vi "Extract_Hex_From_String_Delimited_With_Bytes_LV2015.vi"(8 "error in (no error)":errorcluster, 11 "String":string="1234 56 7 8 9A BC DEF1\nabcdefghijklmnopqrstuvwxyz1234567890\n\nasdfjlkasjdf;lk ajsdovj 239845uj sdklfhjg98bn248vg 9mufy gfalkjdfn" caption="HexString with or without delimitation") -> (0 "error out":errorcluster, 3 "Extracted Hex with delimitation at every byte":string="12 34 56 78 9A BC DE F1 AB CD EF 12 34 56 78 90 AD FA DF AD 23 98 45 DF 98 B2 48 9F FA DF" caption="HexByte delimited string")   [LabVIEW 2015]
panel:
  # "Connector Pane"
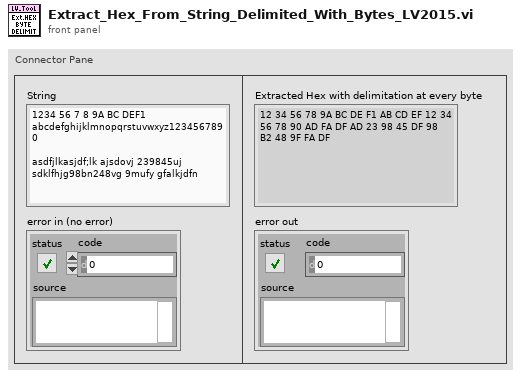
[diagram p1: front panel]
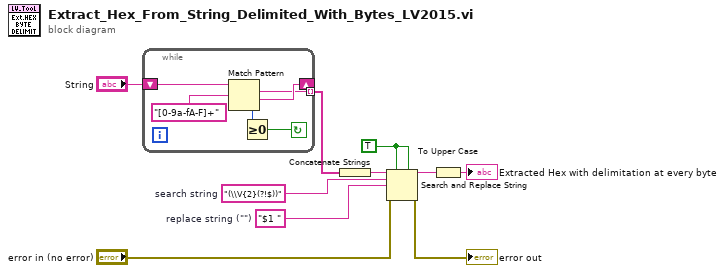
[diagram p0: block diagram]
diagram:
  w7 = TRUE ("replace all? (F)")
  w9 = "$1 "  # replace string ("")
  w10 = "(\\V{2}(?!$))"  # search string
  n1 = while {
    shift-right: [w12] -> _
    shift-left: "String" -> [w16]
    tunnel: [w11] -> w3 mode=indexing
    stop <- w14 continue-if-true
    n2 = Match Pattern(string=w16, regular expression="[0-9a-fA-F]+") -> (match substring=w11:string, after substring=w12:string, offset past match=w15:i32)  [unwired: 2 out]
    n3 = Greater Or Equal To 0?(x=w15) -> (x >= 0?=w14:bool)
  }
  n4 = Concatenate Strings(w3) -> (w2:string)
  n5 = Search and Replace String(replace all?=w7, multiline?=w7, input string=w2, search string=w10, replace string=w9, error in="error in (no error)") -> (result string=w8:string, error out=→"error out":errorcluster)  [unwired: 2 in, 2 out]
  n6 = To Upper Case(1:w8) -> (0:→"Extracted Hex with delimitation at every byte":string)
